vi "CreatePrivateEvents.vi"(8 "error in (no error)":errorcluster, 11 "MAUI":refnum<class "SMO.UI.MAUI.lvclass">) -> (0 "error out":errorcluster, 3 "MAUI out":refnum<class "SMO.UI.MAUI.lvclass">)   [LabVIEW 2016, in "SMO.UI.MAUI.lvclass"]
doc: "---------------------------------------------------------------\nJKI State Machine Objects™\nhttp://jki.net/state-machine-objects/\nCopyright (C) 2005-2015, JKI <info@jki.net>\nALL RIGHTS RESERVEDJKI State Machine Objects (SMO) 1.0.0.4\nJKI - JKI\nCopyright (c) 2015, JKI"
uses:
  SMO.UI.MAUI.lvclass
  Typedefs/PrivateEvents--SMO.UI.MAUI.SetEmbedded.ctl
  <vilib>/Levylab/SMO.UI.Embedded/SMO.UI.Embedded.lvclass
  Typedefs/PrivateEvents--SMO.UI.MAUI.GetEmbedded.ctl
  Typedefs/PrivateEvents--SMO.UI.MAUI.SetPanelData.ctl
  Typedefs/PanelData.ctl
  Typedefs/PrivateEvents--SMO.UI.MAUI.GetPanelData.ctl
  Typedefs/PrivateEvents--SMO.UI.MAUI.UpdatePanel.ctl
  Typedefs/PrivateEvents--SMO.UI.MAUI.PopSubpanel.ctl
  SMO.UI.MAUI.lvclass/SMO.UI.MAUI.ctl
  <vilib>/JKI/JKI SMO/SMO.UI/SMO.UI.lvclass
panel:
  # "For instructions on how to use the JKI State Machine Objects, examples and video tutorials, visit:\nhttp://jki.net/state-machine-objects/\n\nJKI State Machine Objects™\nhttp://jki.net/state-machine-objects/\nCopyright (C) 2005-2015, JKI <info@jki.net>\nALL RIGHTS RESERVED"
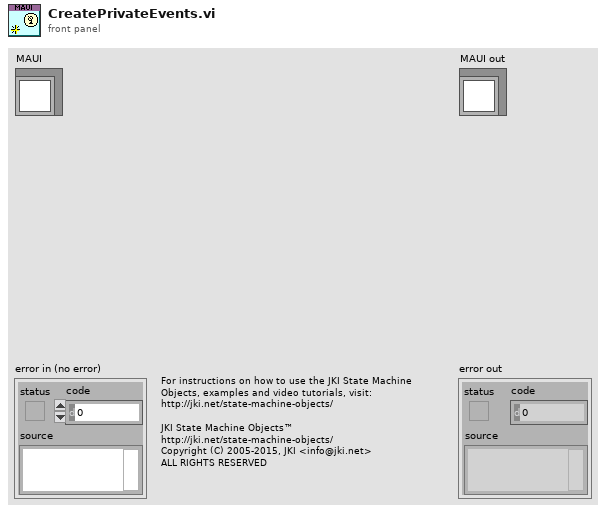
[diagram p1: front panel]
types:
  T1 = typedef "SMO.UI.MAUI.lvclass/PrivateEvents--SMO.UI.MAUI.PopSubpanel.ctl" = i32
  T2 = typedef "SMO.UI.MAUI.lvclass/PrivateEvents--SMO.UI.MAUI.UpdatePanel.ctl" = cluster{"Panel":i32, "Embedded":i32}
  T3 = typedef "SMO.UI.MAUI.lvclass/PrivateEvents--SMO.UI.MAUI.GetPanelData.ctl" = refnum<notifier>
  T4 = typedef "SMO.UI.MAUI.lvclass/PrivateEvents--SMO.UI.MAUI.SetPanelData.ctl" = T5[]
  T5 = typedef "SMO.UI.MAUI.lvclass/PanelData.ctl" = cluster{"SubPanel":refnum<vi>, "Ring":refnum<vi>, "Active":i32}
  T6 = typedef "SMO.UI.MAUI.lvclass/PrivateEvents--SMO.UI.MAUI.GetEmbedded.ctl" = cluster{"notifier out":refnum<notifier>}
  T7 = typedef "SMO.UI.MAUI.lvclass/PrivateEvents--SMO.UI.MAUI.SetEmbedded.ctl" = cluster{"Subpanels":refnum<class "SMO.UI.Embedded.lvclass">[]}
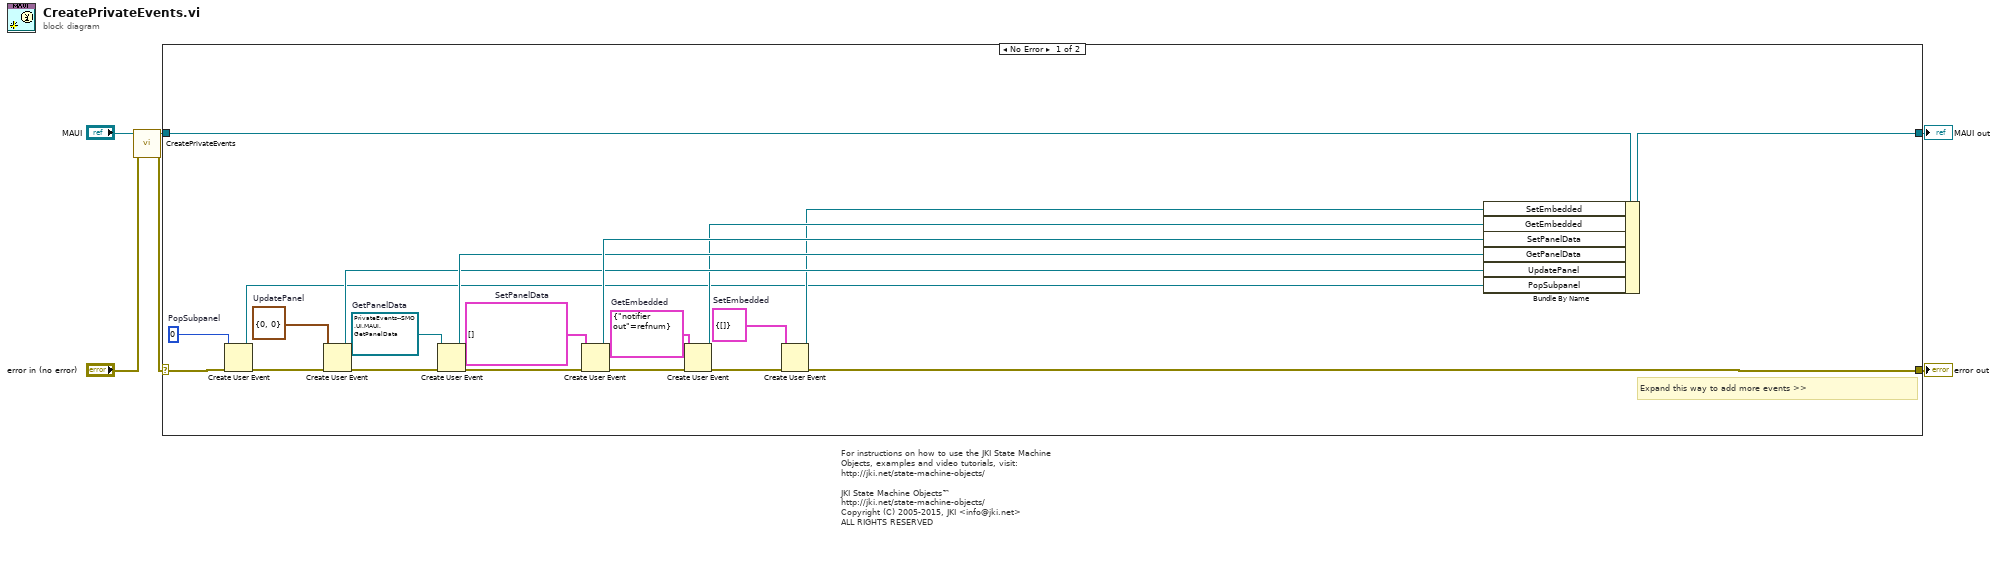
[diagram p0: block diagram]
diagram:
  # "For instructions on how to use the JKI State Machine Objects, examples and video tutorials, visit:\nhttp://jki.net/state-machine-objects/\n\nJKI State Machine Objects™\nhttp://jki.net/state-machine-objects/\nCopyright (C) 2005-2015, JKI <info@jki.net>\nALL RIGHTS RESERVED"
  n1 = call-parent "CreatePrivateEvents.vi"("error in (no error)"="error in (no error)", "SMO.UI"="MAUI") -> ("error out"=w1:errorcluster, "SMO.UI out"=w3:refnum<class "SMO.UI.MAUI.lvclass">)  [unwired: 8 in]
  n2 = case shown="No Error" w1 {
    selector: w1 -> [w26 w29]
    tunnel: [w13 w29] -> w5
    tunnel: [w25 w28] -> w6
    tunnel: w3 -> [w27 w28]
    frame No Error {
      w8 = T1 0  # PopSubpanel
      w15 = T2 {"Panel"=0, "Embedded"=0}  # UpdatePanel
      w18 = T3 refnum  # GetPanelData
      w21 = T4 []  # SetPanelData
      w22 = T6 {"notifier out"=refnum}  # GetEmbedded
      w24 = T7 {"Subpanels"=[]}  # SetEmbedded
      # "Expand this way to add more events >>"
      n3 = Create User Event(user event datatype=w8, error in=w26) -> (user event=w7:refnum<user-event>, error out=w9:errorcluster)
      n4 = Create User Event(user event datatype=w15, error in=w9) -> (user event=w14:refnum<user-event>, error out=w16:errorcluster)
      n5 = Create User Event(user event datatype=w18, error in=w16) -> (user event=w17:refnum<user-event>, error out=w19:errorcluster)
      n6 = Create User Event(user event datatype=w21, error in=w19) -> (user event=w20:refnum<user-event>, error out=w12:errorcluster)
      n7 = Create User Event(user event datatype=w22, error in=w12) -> (user event=w11:refnum<user-event>, error out=w23:errorcluster)
      n8 = Create User Event(user event datatype=w24, error in=w23) -> (user event=w10:refnum<user-event>, error out=w13:errorcluster)
      n9 = Bundle By Name(cluster=w27, "SetEmbedded"=w10, "GetEmbedded"=w11, "SetPanelData"=w20, "GetPanelData"=w17, "UpdatePanel"=w14, "PopSubpanel"=w7) -> (w25:refnum<class "SMO.UI.MAUI.lvclass">)
    }
    frame Error {
    }
  }
  "error out" <- w5
  "MAUI out" <- w6
